vi "Handle Command.vi"(8 "error in (no error)":errorcluster, 9 "Data":variant, 10 "Command":string, 11 "Control Experiment":refnum<class "Control Experiment.lvclass">) -> (0 "error out":errorcluster, 1 "Processed Data":variant, 2 "Command":string, 3 "Control Experiment out":refnum<class "Control Experiment.lvclass">)   [LabVIEW 2016, in "Control Experiment.lvclass"]
uses:
  Control Experiment.lvclass
  <userlib>/LevyLab/Levylab Instruments/SMOs/Instrument/Instrument.lvclass
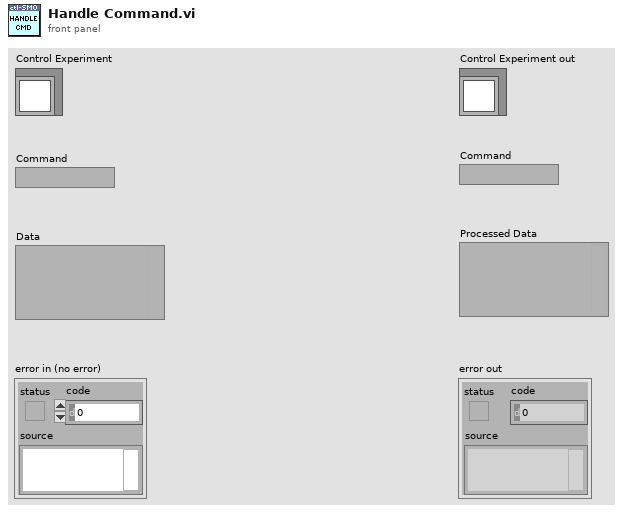
[diagram p1: front panel]
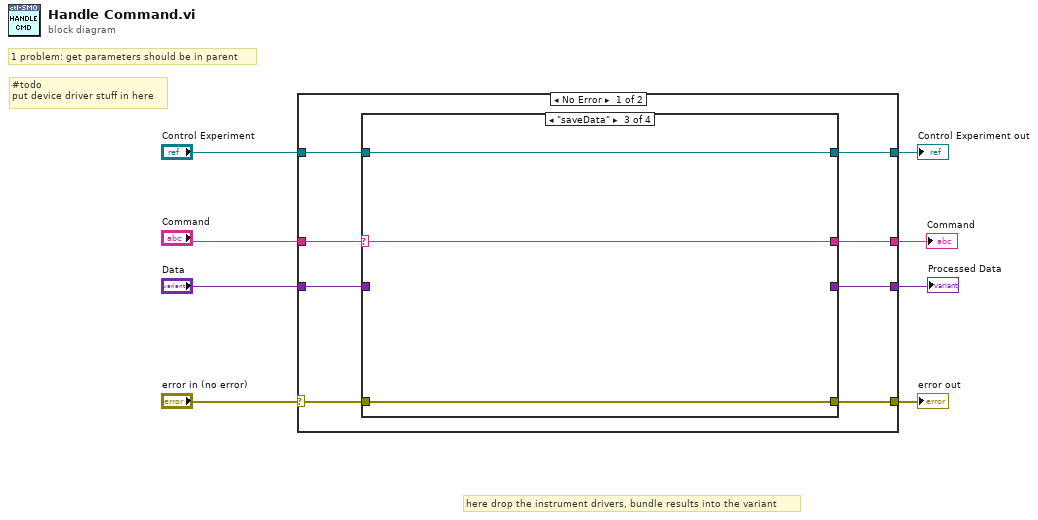
[diagram p0: block diagram]
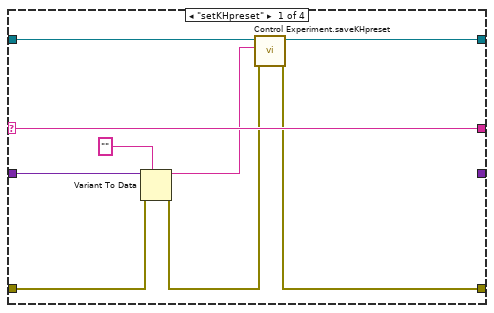
[diagram p2: hidden frame]
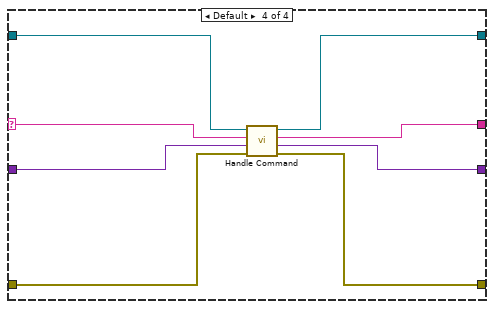
[diagram p4: hidden frame]
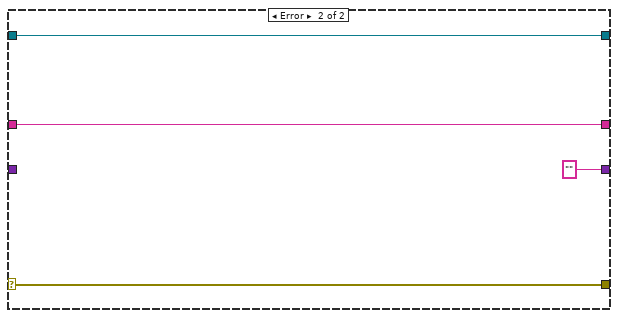
[diagram p5: hidden frame]
diagram:
  # "here drop the instrument drivers, bundle results into the variant"
  # "1 problem: get parameters should be in parent"
  # "#todo\nput device driver stuff in here"
  n1 = case shown="No Error" "error in (no error)" {
    selector: "error in (no error)" -> [w12 w43]
    tunnel: [w10 w43] -> w6
    tunnel: [w14 w42] -> w5
    tunnel: "Control Experiment" -> [w15 w42]
    tunnel: "Command" -> [w16 w40]
    tunnel: [w13 "" ("String")] -> w3
    tunnel: "Data" -> [w11 _]
    tunnel: [w9 w40] -> w1
    frame No Error {
      n2 = case shown="\"saveData\"" w16 {
        selector: w16 -> [w25 w27 w30 w39]
        tunnel: w15 -> [w23 w26 w31 w36]
        tunnel: [w17 w26 w31 w33] -> w14
        tunnel: [_ w26 _ w35] -> w13
        tunnel: w12 -> [w19 w28 w29 w37]
        tunnel: w11 -> [w22 _ _ w38]
        tunnel: [w24 w28 w29 w34] -> w10
        tunnel: [w25 w27 w30 w32] -> w9
        frame "setKHpreset" {
          n3 = Variant To Data(error in=w19, type="", Variant=w22) -> (data=w20:string, error out=w18:errorcluster)
          n4 = call "Control Experiment.saveKHpreset.vi"("error in (no error)"=w18, "saveKHpreset"=w20, "Control Experiment"=w23) -> ("error out"=w24:errorcluster, "Control Experiment out"=w17:refnum<class "Control Experiment.lvclass">)  [unwired: 7 in]
        }
        frame "getXML" {
        }
        frame "saveData" {
        }
        frame Default {
          n5 = call-parent "Handle Command.vi"("error in (no error)"=w37, "Data"=w38, "Command"=w39, "Instrument in"=w36) -> ("error out"=w34:errorcluster, "Processed Data"=w35:variant, "Command"=w32:string, "Instrument out"=w33:refnum<class "Control Experiment.lvclass">)  [unwired: 4 in]
        }
      }
    }
    frame Error {
    }
  }
  "error out" <- w6
  "Control Experiment out" <- w5
  "Command" <- w1
  "Processed Data" <- w3
